vi "ExSubAsyncColDispStrPhoto.vi"(2 "error in (no error)":errorcluster, 3 "Store Data":bool, 4 "Display Title":string, 5 "Handle Cluster":T1) -> (0 "error out":errorcluster, 1 "Handle Cluster Out":T1)   [LabVIEW 2010]
panel:
  # "ExSubAsyncColDispStr:\nThis Sub-VI does the data \ncollection, display, and storage \nfor Async camera operations."
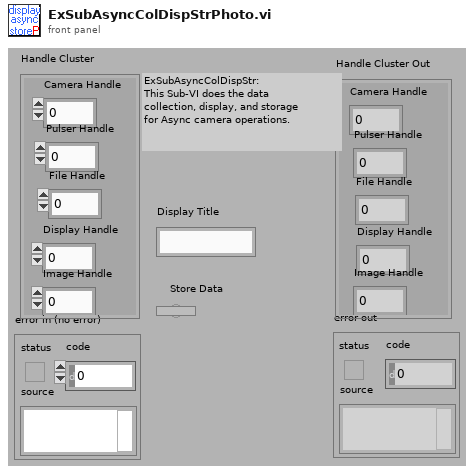
[diagram p1: front panel]
types:
  T1 = cluster{"Camera Handle":u32, "Pulser Handle":u32, "File Handle":u32, "Display Handle":u32, "Image Handle":u32}
  T2 = cluster{"Camera Handle":u32, "Pulser Handle":u32, "File Handle":u32, "Display Handle":u32, "Data Handle":u32}
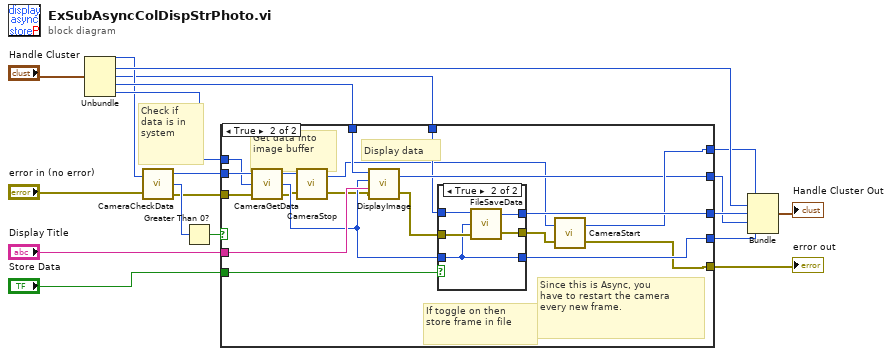
[diagram p0: block diagram]
diagram:
  # "Check if \ndata is in\nsystem"
  n1 = Unbundle("Handle Cluster") -> ("Camera Handle"=w6:u32, "Pulser Handle"=w9:u32, "File Handle"=w1:u32, "Display Handle"=w11:u32, "Image Handle"=w12:u32)
  n2 = call <userlib>:"CameraCheckData.vi"("Camera Handle"=w6, "error in"="error in (no error)") -> ("Camera Handle"=w16:u32, "Number Of Frames Available"=w15:i32, "error out"=w14:errorcluster)
  n3 = Greater Than 0?(x=w15) -> (x > 0?=w17:bool)
  n4 = case shown="True" w17 {
    tunnel: w16 -> [w24 w43]
    tunnel: w14 -> [w23 w42]
    tunnel: w12 -> [w21 w40]
    tunnel: w11 -> [w22 w39]
    tunnel: [w24 w31] -> w7
    tunnel: [w20 w41] -> w5
    tunnel: "Display Title" -> [_ w38]
    tunnel: w1 -> [w20 w29]
    tunnel: [w22 w30] -> w4
    tunnel: [w23 w32] -> w8
    tunnel: [w21 w36] -> w3
    tunnel: "Store Data" -> [_ w35]
    frame False {
    }
    frame True {
      # "If toggle on then\nstore frame in file"
      # "Since this is Async, you\nhave to restart the camera\nevery new frame."
      # "Display data"
      # "Get data into\nimage buffer"
      n5 = call <userlib>:"CameraGetData.vi"("error in"=w42, "Data Handle"=w40, "Camera Handle"=w43) -> ("error out"=w28:errorcluster, "Data Handle"=w37:u32, "Camera Handle"=w27:u32)
      n6 = call <userlib>:"CameraStop.vi"("error in"=w28, "Camera Handle"=w27) -> ("error out"=w25:errorcluster, "Camera Handle"=w26:u32)
      n7 = call <userlib>:"DisplayImage.vi"("error in"=w25, "Title"=w38, "Image Handle"=w37, "Display Handle"=w39) -> ("error out"=w34:errorcluster, "Display Handle"=w30:u32)
      n8 = case shown="True" w35 {
        tunnel: [w46 w51] -> w41
        tunnel: w34 -> [w45 w50]
        tunnel: w29 -> [w46 w47]
        tunnel: [w45 w49] -> w33
        tunnel: w37 -> [w44 w48]
        tunnel: [w44 w48] -> w36
        frame False {
        }
        frame True {
          n9 = call <userlib>:"FileSaveData.vi"("error in"=w50, "Image Handle"=w48, "File Handle"=w47) -> ("error out"=w49:errorcluster, "File Handle"=w51:u32)
        }
      }
      n10 = call <userlib>:"CameraStart.vi"("error in"=w33, "Camera Handle"=w26) -> ("error out"=w32:errorcluster, "Camera Handle"=w31:u32)
    }
  }
  "error out" <- w8
  n11 = Bundle("Camera Handle"=w7, "Pulser Handle"=w9, "File Handle"=w5, "Display Handle"=w4, "Data Handle"=w3) -> (→"Handle Cluster Out":T2)  [unwired: 1 in]
